vi "二维码打印.vi"() -> ()   [LabVIEW 2013]
uses:
  <vilib>/Utility/miscctls.llb/LVBoundsTypeDef.ctl
panel:
  out "error out":errorcluster
  out "Status":i8
  in  "rect":T1
  in  "error in (no error)":errorcluster
  out "new picture":picture caption="新图片"
  in  "String":string
  in  "布尔":bool
  in  "QrCodeImgControl":refnum<k24>(container)
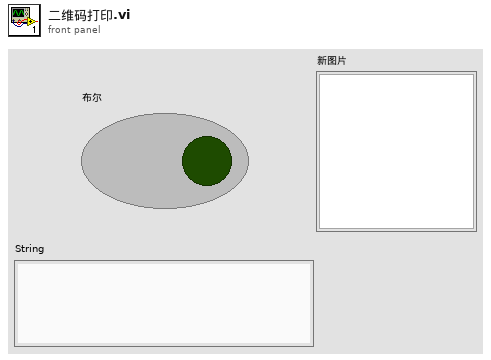
[diagram p1: front panel]
types:
  T1 = cluster{"left":i16, "top":i16, "right":i16, "bottom":i16}
  T2 = typedef "LVBoundsTypeDef.ctl" = cluster{"Width":u32, "Height":u32}
  T3 = typedef "imagedata.ctl" = cluster{"image type":i32, "image depth":i32, "image":u8[], "mask":u8[], "colors":u32[], "Rectangle":cluster{"left":i16, "top":i16, "right":i16, "bottom":i16}}
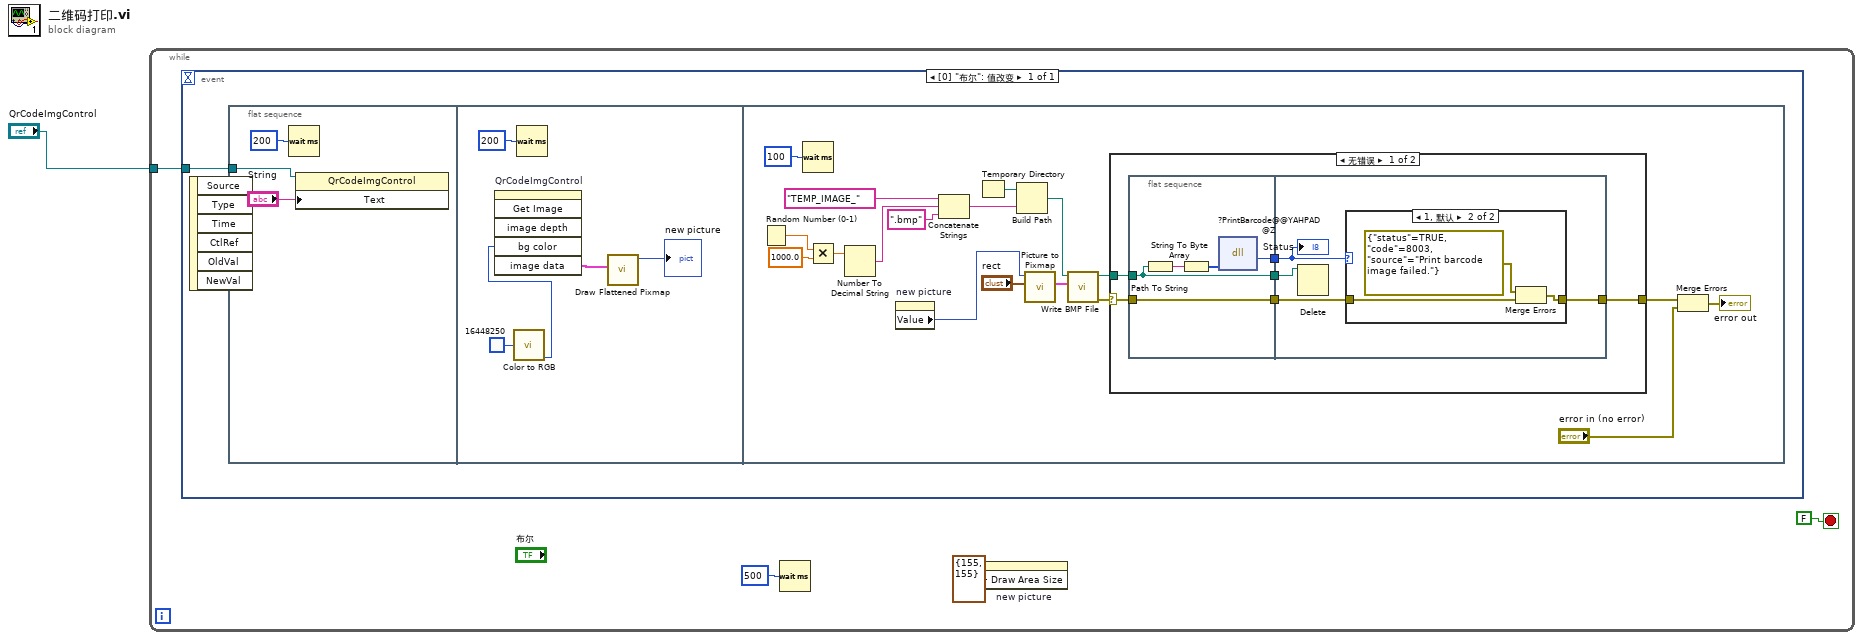
[diagram p0: block diagram]
diagram:
  n1 = while {
    tunnel: "QrCodeImgControl" -> [w5]
    stop <- FALSE stop-if-true
    n2 = event shown="[0] \"布尔\": 值改变" {
      selector: _ -> [_]
      dyn-events: _ -> [_]
      timeout: _ -> [_]
      tunnel: w5 -> [w6]
      event "布尔": Value Change {
        n3 = event-data() -> ()  [unwired: 1 in, 6 out]
        n4 = flat-sequence {
          tunnel: w6 -> [w9]
          frame #0 {
            n5 = Wait (ms)(milliseconds to wait=u32 200 ("等待时间（毫秒）")) -> ()  [unwired: 1 out]
            n6 = property class="QrCodeImgControl"(reference=w9, "Text"="String") -> ()  [unwired: 1 in, 2 out]
          }
          frame #1 {
            n7 = call <vilib>:"Color to RGB.vi"("Color"=u32 16448250) -> ("B"=w11:u8)  [unwired: 3 out]
            n8 = invoke on="QrCodeImgControl" class="AXCont" method="Get Image"("bg color"=w11) -> ("image data"=w14:T3)  [unwired: 5 in, 5 out]
            n9 = Wait (ms)(milliseconds to wait=u32 200 ("等待时间（毫秒）")) -> ()  [unwired: 1 out]
            n10 = call <vilib>:"Draw Flattened Pixmap.vi"("image data"=w14) -> ("new picture"=→"new picture":picture)  [unwired: 8 in]
          }
          frame #2 {
            n11 = Random Number (0-1)() -> (number: 0 to 1=w25:dbl)
            n12 = Wait (ms)(milliseconds to wait=u32 100 ("等待时间（毫秒）")) -> ()  [unwired: 1 out]
            n13 = Multiply(x=w25, y=1000.0) -> (x*y=w26:dbl)
            n14 = Number To Decimal String(number=w26) -> (decimal integer string=w27:string)  [unwired: 1 in]
            n15 = property on="new picture" class="Pict"() -> ("Value"=w16:picture)  [unwired: 2 in, 2 out]
            n16 = Concatenate Strings("TEMP_IMAGE_", w27, ".bmp") -> (w28:string)
            n17 = Temporary Directory() -> (w21:path)
            n18 = Build Path(base path=w21, name or relative path=w28) -> (appended path=w22:path)
            n19 = call <vilib>:"Picture to Pixmap.vi"("rect"="rect", "picture"=w16) -> ("image data"=w20:T3)  [unwired: 8 in, 1 out]
            n20 = call <vilib>:"Write BMP File.vi"("image data"=w20, "path to BMP file"=w22) -> ("error out"=w24:errorcluster, "path"=w23:path)  [unwired: 8 in]
            n21 = case shown="无错误" w24 {
              selector: w24 -> [w35 w52]
              tunnel: w23 -> [w38 _]
              tunnel: [w33 w52] -> w30
              frame No Error {
                n22 = flat-sequence {
                  tunnel: w38 -> [w40]
                  tunnel: [w43] -> w37
                  tunnel: [w40] -> w36
                  tunnel: w35 -> [w39]
                  tunnel: [w39] -> w34
                  tunnel: w37 -> [w46]
                  tunnel: w36 -> [w47]
                  tunnel: w34 -> [w45]
                  tunnel: [w44] -> w33
                  frame #0 {
                    n23 = Path To String(path=w40) -> (string=w42:string)
                    n24 = String To Byte Array(string=w42) -> (unsigned byte array=w41:u8[])
                    n25 = dll-call lib="PTH1\\abs F智能扦样机摄像头储存与回放\t条码库Src\tLVBarcode\nLVBarcode.dll" fn="?PrintBarcode@@YAHPAD@Z"("FileName"=w41) -> ("返回类型"=w43:i8)  [unwired: 4 in, 2 out]
                  }
                  frame #1 {
                    n26 = Delete(path (use dialog)=w47) -> ()  [unwired: 4 in, 3 out]
                    n27 = case shown="1, 默认" w46 {
                      tunnel: w45 -> [w48 w51]
                      tunnel: [w48 w49] -> w44
                      frame 0 {
                      }
                      frame 1, Default {
                        n28 = Merge Errors(errorcluster {"status"=TRUE, "code"=8003, "source"="Print barcode image failed."} ("input cluster"), w51) -> (w49:errorcluster)
                      }
                    }
                    "Status" <- w46
                  }
                }
              }
              frame Error {
              }
            }
            n29 = Merge Errors(w30, "error in (no error)") -> (→"error out":errorcluster)
          }
        }
      }
    }
    n30 = Wait (ms)(milliseconds to wait=u32 500 ("等待时间（毫秒）")) -> ()  [unwired: 1 out]
    n31 = property on="new picture" class="Pict"("Draw Area Size"=T2 {"Width"=155, "Height"=155} ("绘图区域大小")) -> ()  [unwired: 2 in, 2 out]
  }
